vi "Add Timing Channels RTM.vi"(8 "error in (no error)":errorcluster, 11 "Node Ptr":T1 format="%.0x") -> (0 "error out":errorcluster)   [LabVIEW 2024, in "AIM ARINC 429 System Explorer.lvlib"]
uses:
  AIM ARINC 429 System Explorer.lvlib
  Includes/AIM ARINC 429 System Explorer.lvlibp/1abvi3w/vi.lib/NI VeriStand/Custom Device API/Custom Device Item Ref.ctl
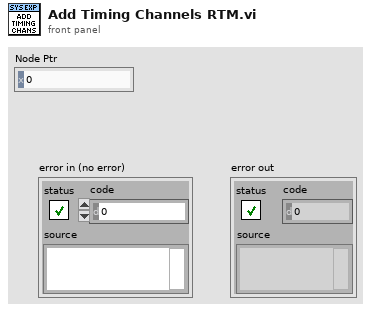
[diagram p1: front panel]
types:
  T1 = typedef "AIM ARINC 429 System Explorer.lvlibp/Custom Device API.lvlib/Custom Device Item Ref.ctl" = u64
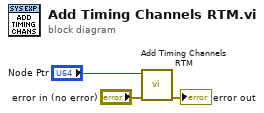
[diagram p0: block diagram]
diagram:
  n1 = call "Add Timing Channels RTM.vi"("error in"="error in (no error)", "Node Ptr"="Node Ptr") -> ("error out"=→"error out":errorcluster)  [unwired: 9 in]
